vi "Pump Settings Dialog.vi"(8 "error in (no error)":errorcluster, 10 "Message Queues":T15, 11 "Pump Module State Cluster In":T1={"Pump Module Config"={"GUID"="", "Drop Coords"={"Horizontal"=0, "Vertical"=0}, "Process Name"="", "Queue Name"="", "Settings"={"Cycle Period"=500.0, "Ismatech"={"VISA resource name"="", "Simulated?"=TRUE, "Pump Number"=1.0, "Reverse?"=FALSE}, "Masterflex"={"VISA resource name"="", "Simulated?"=TRUE, "Pump Number"=1.0, "Reverse?"=FALSE}, "Manual Entry"=0.0, "VICI Settings"={"VISA resource name"="", "Simulated?"=TRUE, "Pump Letter"="", "Reverse?"=FALSE}, "Output Device"=enum."Default", "Tacmina Settings"={"Analog DAQ Task"="", "Digital DAQ Task"=""}, "KNF SIMDOS Settings"={"VISA resource name"="", "Simulated?"=TRUE}, "ASIA Pump C"={"ASIA Pump #"=0, "channel"=0, "Simulated"=FALSE}, "FLOM Settings"={"VISA resource name"="", "Simulated?"=TRUE, "Pump Number"=0.0}, "Pump Calibration File"=path "", "Calibration Slope"=0.0, "Calibration Y Intercept"=0.0, "Pump Cal Enum"=0, "SSI PR Settings"={"VISA resource name"="", "Simulated?"=FALSE}}, "Load Count"=0}, "State"=enum."Idle", "Start Time"=timestamp(0 s since 1904-01-01), "Current Time"=timestamp(0 s since 1904-01-01), "First Iteration"=FALSE, "Data"={"Pump Speed"=0.0}, "Process Name"="", "Pump On?"=FALSE} {"Pump Module Config"."Settings"."ASIA Pump C"."channel" min=0 max=1 step=1; "Pump Module Config"."Settings"."Masterflex"."Pump Number" min=1.0 max=20.0 step=1.0; "Pump Module Config"."Settings"."Ismatech"."Pump Number" min=1.0 max=20.0 step=1.0}) -> (0 "error out":errorcluster, 1 "Cancelled?":bool=TRUE, 2 "UI Refresh Needed?":bool, 3 "Pump Module Config Out":T2={"GUID"="", "Drop Coords"={"Horizontal"=0, "Vertical"=0}, "Process Name"="", "Queue Name"="", "Settings"={"Cycle Period"=0.0, "Ismatech"={"VISA resource name"="", "Simulated?"=FALSE, "Pump Number"=0.0, "Reverse?"=FALSE}, "Masterflex"={"VISA resource name"="", "Simulated?"=FALSE, "Pump Number"=0.0, "Reverse?"=FALSE}, "Manual Entry"=0.0, "VICI Settings"={"VISA resource name"="", "Simulated?"=FALSE, "Pump Letter"="", "Reverse?"=FALSE}, "Output Device"=enum."Default", "Tacmina Settings"={"Analog DAQ Task"="", "Digital DAQ Task"=""}, "KNF SIMDOS Settings"={"VISA resource name"="", "Simulated?"=TRUE}, "ASIA Pump C"={"ASIA Pump #"=0, "channel"=0, "Simulated"=FALSE}, "FLOM Settings"={"VISA resource name"="", "Simulated?"=TRUE, "Pump Number"=0.0}, "Pump Calibration File"=path "", "Calibration Slope"=0.0, "Calibration Y Intercept"=0.0, "Pump Cal Enum"=0, "SSI PR Settings"={"VISA resource name"="", "Simulated?"=FALSE}}, "Load Count"=0} {"Settings"."ASIA Pump C"."channel" min=0 max=1 step=1; "Settings"."Masterflex"."Pump Number" min=1.0 max=20.0 step=1.0; "Settings"."Ismatech"."Pump Number" min=1.0 max=20.0 step=1.0})   [LabVIEW 2018, in "Pump Module.lvlib"]
doc: "Dialog for selecting user specified settings."
uses:
  Pump Module.lvlib
  Settings/Settings.lvlib
  support/Support Library.lvlib
  Masterflex 7550-30/Masterflex 7550-30.lvlib
  Ismatec ISM 831C/Ismatec ISM 831C.lvlib
  Tacmina QI/Tacmina QI.lvlib
  KNF Pump/KNF SIMDOS.lvlib
  VICI M50 Party Mode/VICI M50 Party Mode.lvlib
  support/Message Queue/Message Queue.lvlib
  support/Message Queue/Enqueue Message (Single).vi
  FLOM Pump/FLOM Pump.lvlib
  SSI PR Class/SSI PR Pump.lvlib
  Measure Instrument/PID 2 Output Enum.ctl
  <vilib>/Utility/xml.llb/Write to XML File(string).vi
  <vilib>/Utility/file.llb/Read Delimited Spreadsheet (string).vi
  Ismatec ISM 831C/Controls/Ismatech Settings Cluster.ctl
  Masterflex 7550-30/Controls/Settings Cluster.ctl
  <vilib>/Utility/miscctls.llb/LVPoint32TypeDef.ctl
  Pump Module Settings Cluster.ctl
  Pump Module Config Cluster.ctl
  support/Message Queue/Message Cluster.ctl
  All Message Queues.ctl
  Tacmina QI/Tacmina QI DAQ Setting.ctl
  Measure Instrument/State Enum.ctl
  Measure Instrument/Feed Module Engine.lvlib
  Pump Module State Cluster.ctl
  KNF Pump/Settings Cluster plus SIMDOS.ctl
  ASIA Pump/Pump Settings.ctl
  ASIA Pump.lvlib
  VICI M50 Party Mode/Settings Cluster.ctl
  FLOM Pump/Settings Cluster.ctl
  SSI PR Class/SSI PR Settings Cluster.ctl
panel:
  in  "Module Name":string
  out "FLOM VISA Chosen":bool
  out "FLOM Number Chosen":bool
  in  "Pump Settings":T16={"Pump Configuration"={"Cycle Period"=500.0, "Ismatech"={"VISA resource name"="", "Simulated?"=FALSE, "Pump Number"=1.0, "Reverse?"=FALSE}, "Masterflex"={"VISA resource name"="", "Simulated?"=FALSE, "Pump Number"=1.0, "Reverse?"=FALSE}, "Pump %"=0.0, "VICI Settings"={"VISA resource name"="", "Simulated?"=FALSE, "Pump Letter"="", "Reverse?"=FALSE}, "Output Device"=enum."Default", "Tacmina Settings"={"Analog DAQ Task"="", "Digital DAQ Task"=""}, "KNF SIMDOS Settings"={"VISA resource name"="", "Simulated?"=FALSE}, "ASIA Pump C"={"ASIA Pump #"=-1, "channel"=-1, "Simulated"=FALSE}, "FLOM Settings"={"VISA resource name"="", "Simulated?"=FALSE, "Pump Number"=1.0}, "Pump Calibration"=0, "SSI PR Settings"={"VISA resource name"="", "Simulated?"=FALSE}}, "Stop"=FALSE, "Start"=FALSE} {"Pump Configuration"."ASIA Pump C"."channel" min=-1 max=1 step=1; "Pump Configuration"."Ismatech"."Pump Number" min=1.0 max=20.0 step=1.0; "Pump Configuration"."Masterflex"."Pump Number" min=1.0 max=20.0 step=1.0}
  in  "Cancel Button":bool
  in  "OK Button":bool
  # "Non visible portion of dialog (needed for connector pane)."
  # "Output Instruments"
  # "Output Instruments"
  # "Output Instruments"
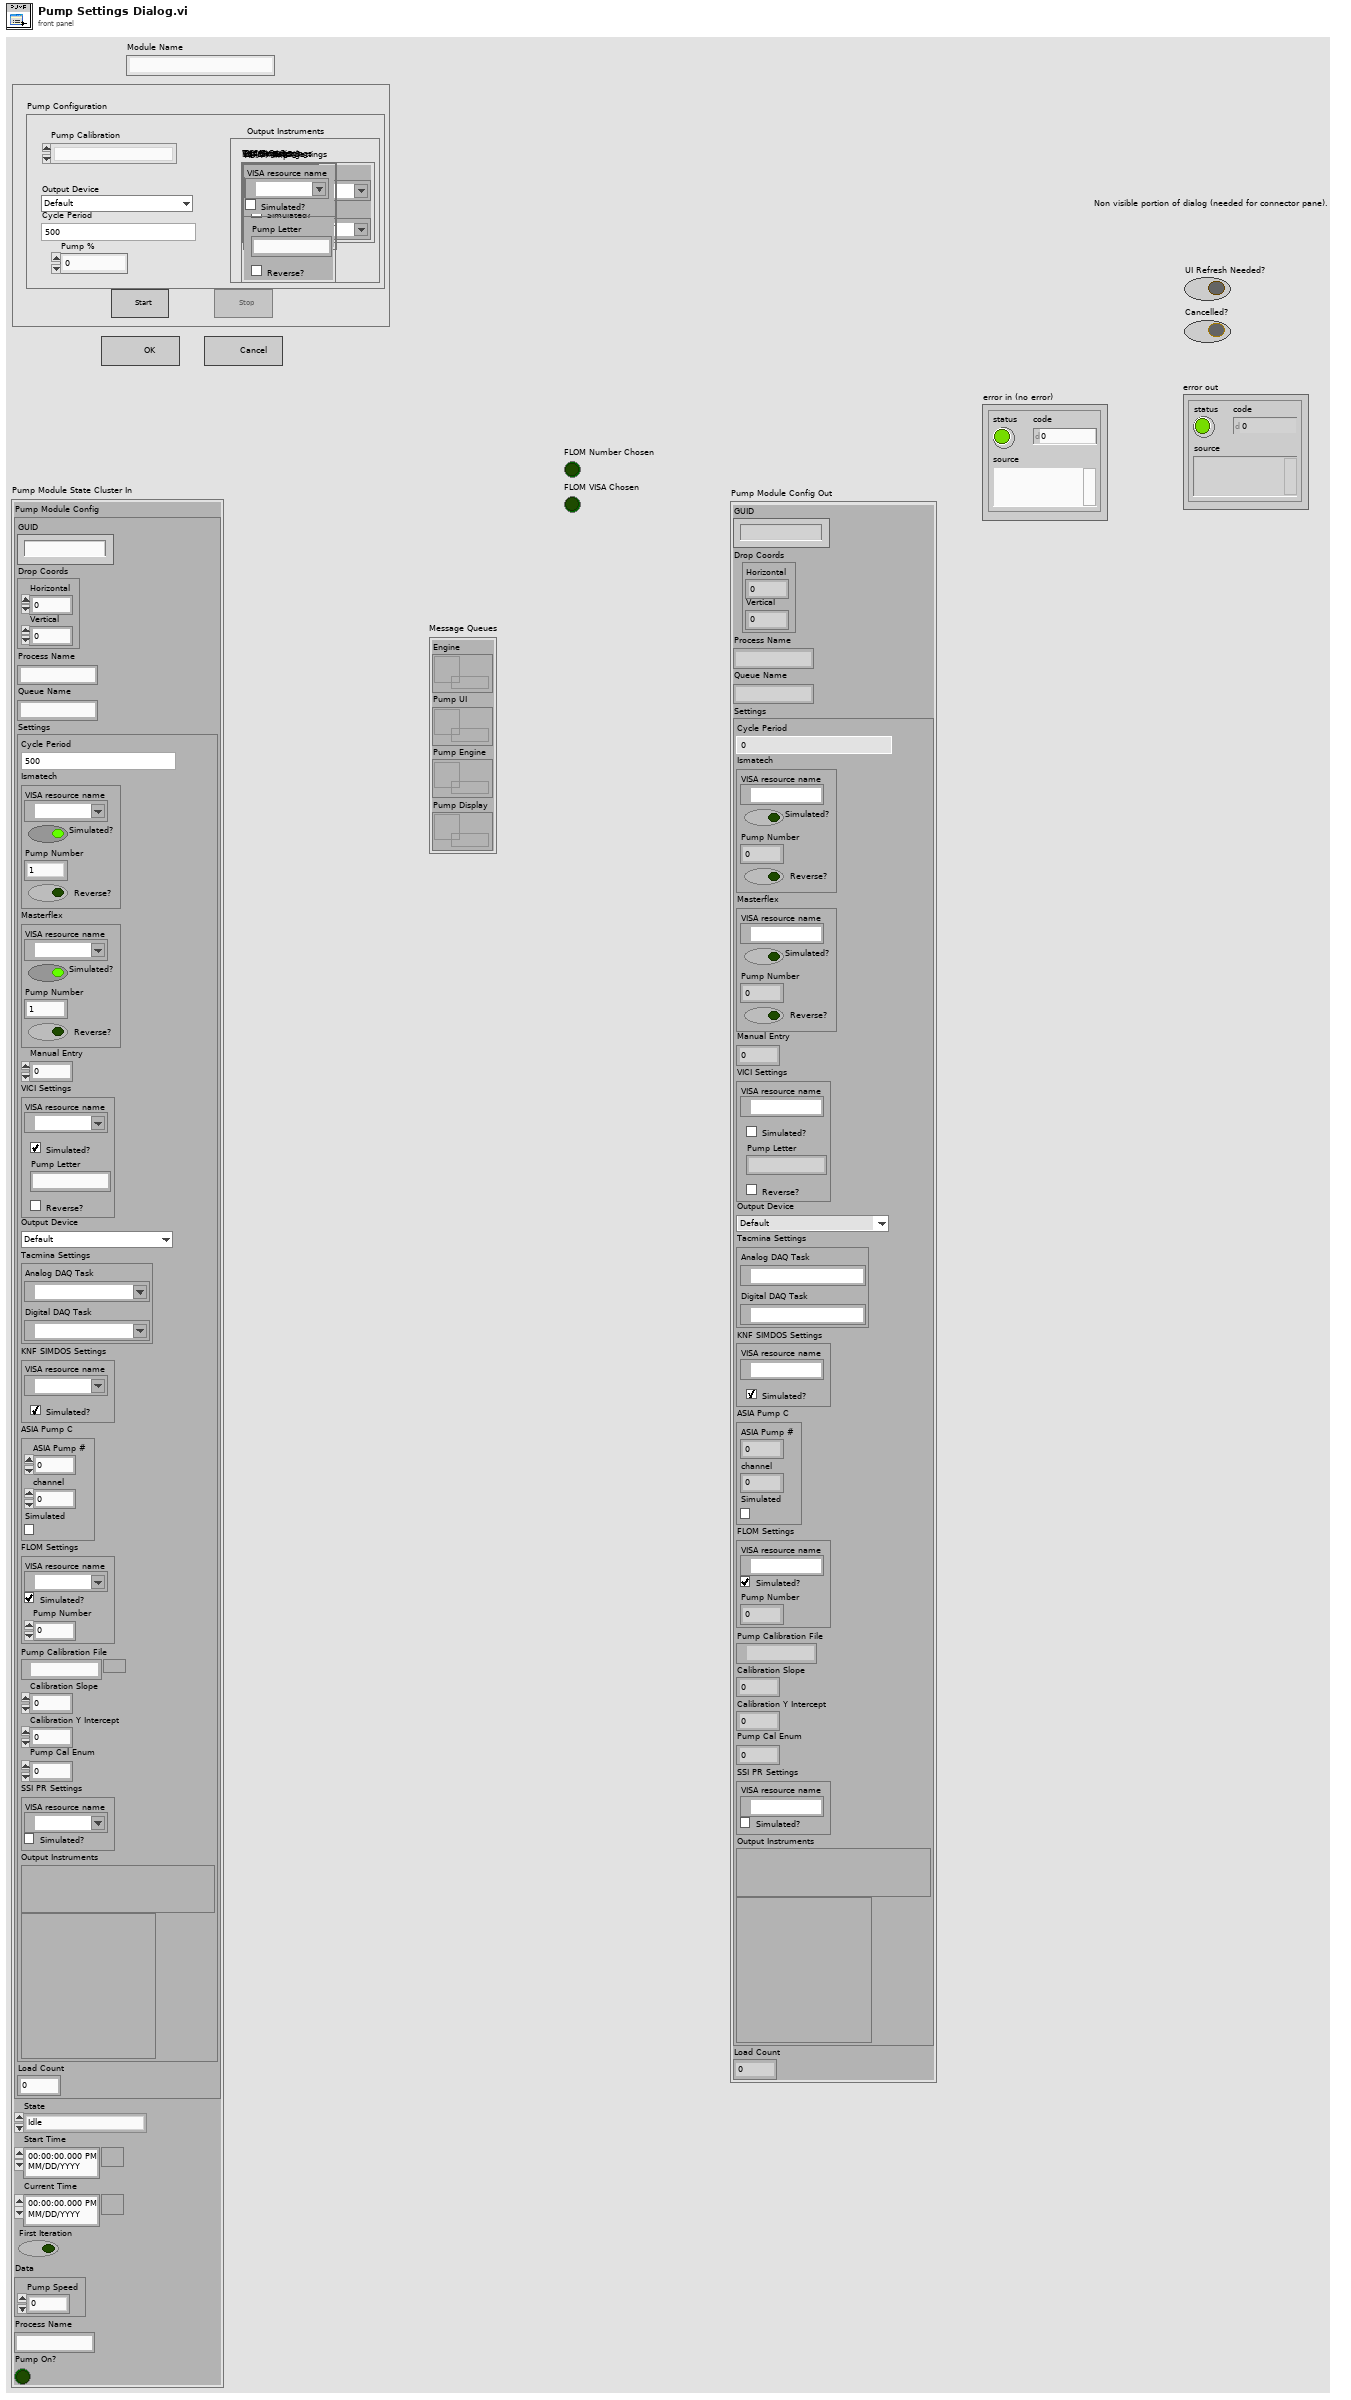
[diagram p1: front panel]
types:
  T1 = typedef "Pump Module.lvlib/Pump Module State Cluster.ctl" = cluster{"Pump Module Config":T2, "State":T14, "Start Time":timestamp, "Current Time":timestamp, "First Iteration":bool, "Data":cluster{"Pump Speed":dbl}, "Process Name":string, "Pump On?":bool}
  T2 = typedef "Pump Module.lvlib/Pump Module Config Cluster.ctl" = cluster{"GUID":string, "Drop Coords":T3, "Process Name":string, "Queue Name":string, "Settings":T4, "Load Count":i32}
  T3 = typedef "LVPoint32TypeDef.ctl" = cluster{"Horizontal":i32, "Vertical":i32}
  T4 = typedef "Pump Module.lvlib/Pump Module Settings Cluster.ctl" = cluster{"Cycle Period":dbl, "Ismatech":T5, "Masterflex":T6, "Manual Entry":dbl, "VICI Settings":T7, "Output Device":T8, "Tacmina Settings":T9, "KNF SIMDOS Settings":T10, "ASIA Pump C":T11, "FLOM Settings":T12, "Pump Calibration File":path, "Calibration Slope":dbl, "Calibration Y Intercept":dbl, "Pump Cal Enum":u16, "SSI PR Settings":T13}
  T5 = typedef "Ismatec ISM 831C.lvlib/Ismatech Settings Cluster.ctl" = cluster{"VISA resource name":refnum<visa-resource-name>, "Simulated?":bool, "Pump Number":dbl, "Reverse?":bool}
  T6 = typedef "Masterflex 7550-30.lvlib/Settings Cluster.ctl" = cluster{"VISA resource name":refnum<visa-resource-name>, "Simulated?":bool, "Pump Number":dbl, "Reverse?":bool}
  T7 = typedef "VICI M50 Party Mode.lvlib/Settings Cluster.ctl" = cluster{"VISA resource name":refnum<visa-resource-name>, "Simulated?":bool, "Pump Letter":string, "Reverse?":bool}
  T8 = typedef "PID 2 Output Enum.ctl" = enum16{"Default", "Ismatec ISM 831C", "Masterflex 7550-30", "VICI", "Tacmina QI", "KNF SIMDOS", "ASIA Type C", "FLOM UI-22-11", "SSI PR"}
  T9 = typedef "Tacmina QI.lvlib/Tacmina QI DAQ Setting.ctl" = cluster{"Analog DAQ Task":refnum<k21>, "Digital DAQ Task":refnum<k21>}
  T10 = typedef "KNF SIMDOS.lvlib/Settings Cluster plus SIMDOS.ctl" = cluster{"VISA resource name":refnum<visa-resource-name>, "Simulated?":bool}
  T11 = typedef "ASIA Pump.lvlib/Pump Settings.ctl" = cluster{"ASIA Pump #":i32, "channel":i32, "Simulated":bool}
  T12 = typedef "FLOM Pump.lvlib/Settings Cluster.ctl" = cluster{"VISA resource name":refnum<visa-resource-name>, "Simulated?":bool, "Pump Number":dbl}
  T13 = typedef "SSI PR Pump.lvlib/SSI PR Settings Cluster.ctl" = cluster{"VISA resource name":refnum<visa-resource-name>, "Simulated?":bool}
  T14 = typedef "Feed Module.lvlib/Feed Module Engine.lvlib/State Enum.ctl" = enum16{"Measuring", "Idle", "Paused"}
  T15 = typedef "Pump Module.lvlib/All Message Queues.ctl" = cluster{"Engine":refnum<queue>, "Pump UI":refnum<queue>, "Pump Engine":refnum<queue>, "Pump Display":refnum<queue>}
  T16 = cluster{"Pump Configuration":cluster{"Cycle Period":dbl, "Ismatech":T5, "Masterflex":T6, "Pump %":dbl, "VICI Settings":T7, "Output Device":T8, "Tacmina Settings":T9, "KNF SIMDOS Settings":T10, "ASIA Pump C":T11, "FLOM Settings":T12, "Pump Calibration":u16, "SSI PR Settings":T13}, "Stop":bool, "Start":bool}
  T17 = enum8{"Enabled", "Disabled", "Disabled and Grayed Out"}
  T18 = typedef "VICI M6 M50 Party Mode.lvlib/Settings Cluster.ctl" = cluster{"VISA resource name":refnum<visa-resource-name>, "Simulated?":bool, "Pump Letter":string, "Reverse?":bool}
  T19 = cluster{"Cycle Period":dbl, "Ismatech":T5, "Masterflex":T6, "Pump %":dbl, "VICI Settings":T18, "Output Device":T8, "Tacmina Settings":T9, "KNF SIMDOS Settings":T10, "ASIA Pump C":T11, "FLOM Settings":T12, "Pump Calibration":u16, "SSI PR Settings":T13}
  T20 = cluster{"Cycle Period":dbl, "Ismatech":T5, "Masterflex":T6, "Pump %":dbl, "VICI Settings":T7, "Output Device":T8, "Tacmina Settings":T9, "KNF SIMDOS Settings":T10, "ASIA Pump C":T11, "FLOM Settings":T12, "Pump Calibration":u16, "SSI PR Settings":T13}
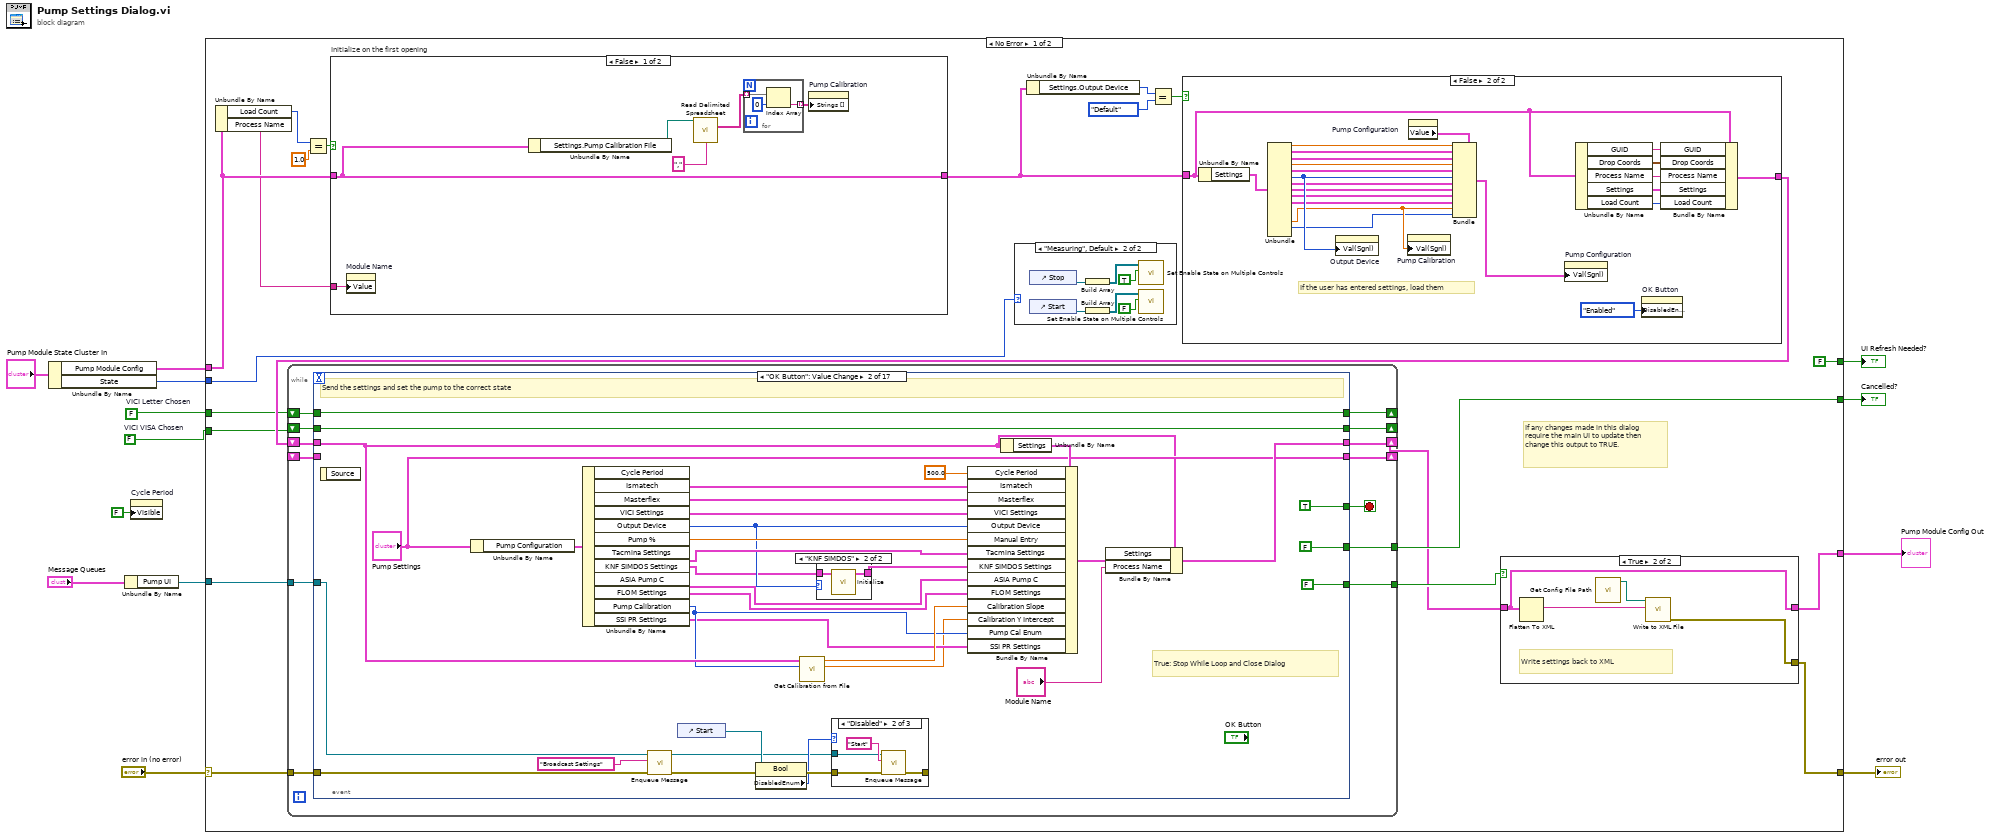
[diagram p0: block diagram]
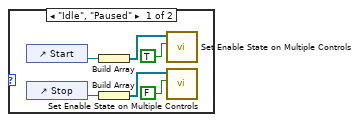
[diagram p2: hidden frame]
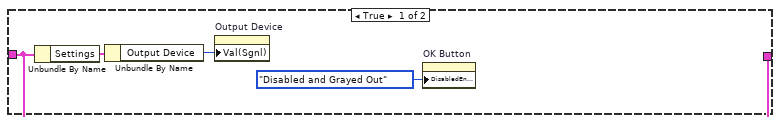
[diagram p3: hidden frame]
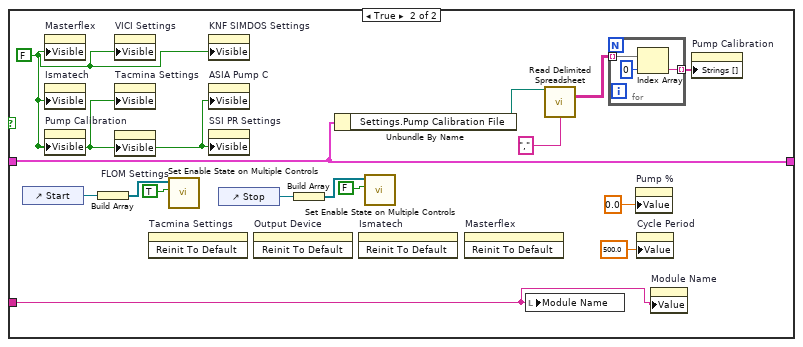
[diagram p4: hidden frame]
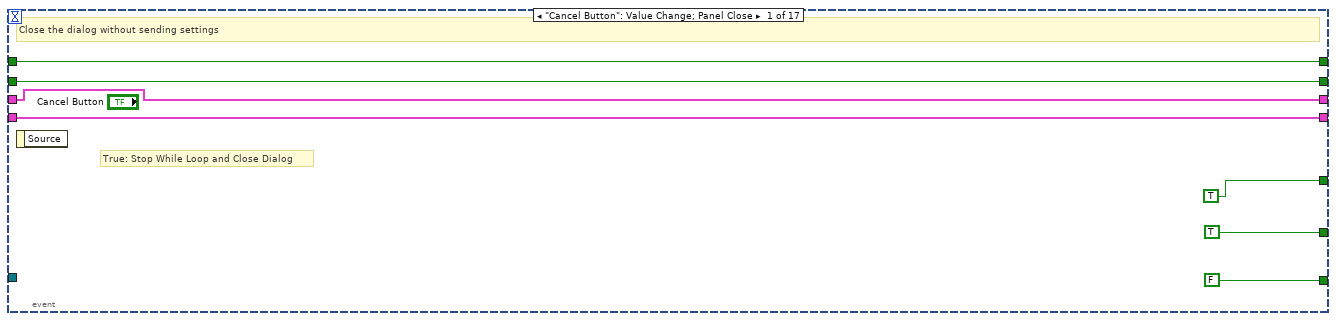
[diagram p5: hidden frame]
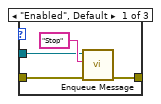
[diagram p6: hidden frame]
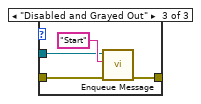
[diagram p7: hidden frame]
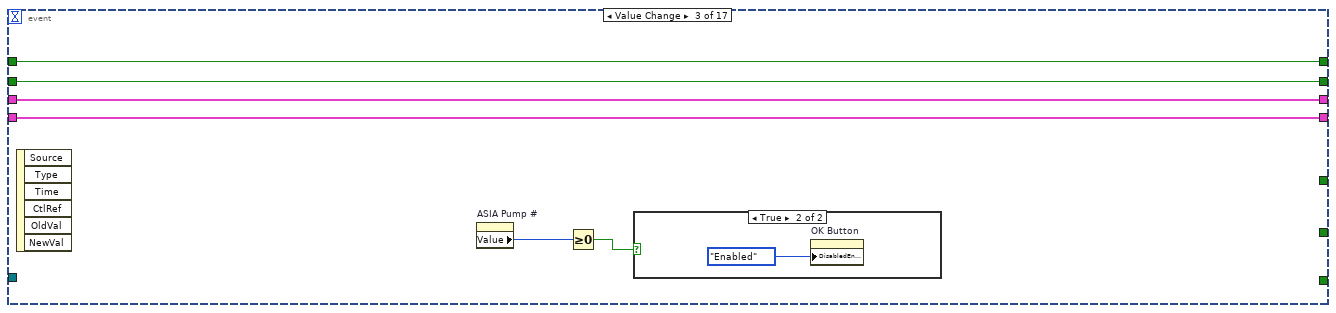
[diagram p9: hidden frame]
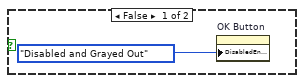
[diagram p10: hidden frame]
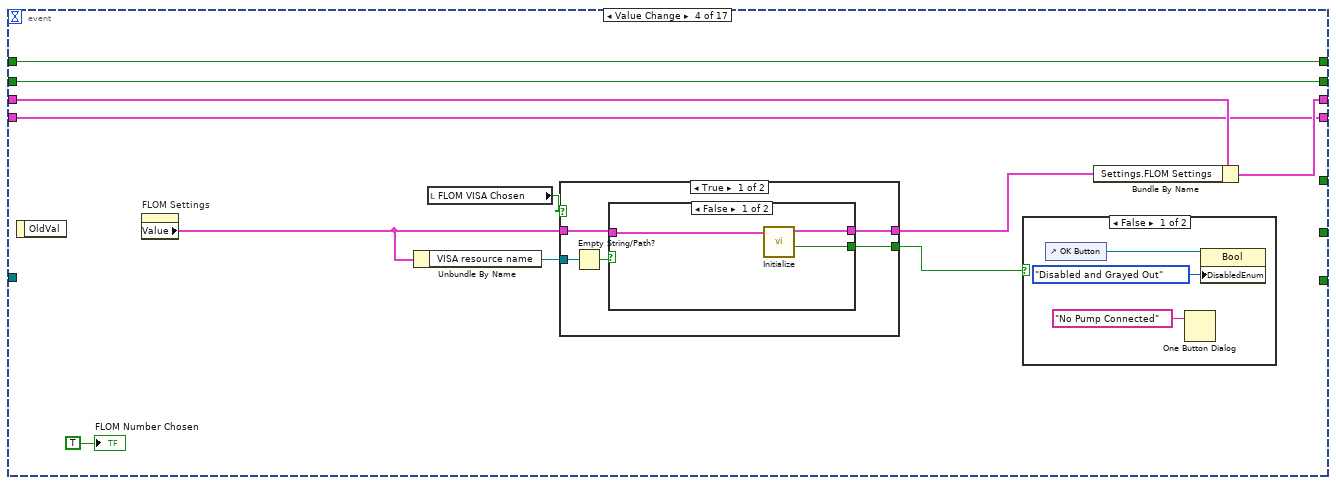
[diagram p11: hidden frame]
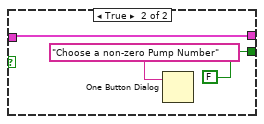
[diagram p12: hidden frame]
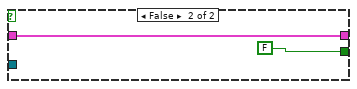
[diagram p13: hidden frame]
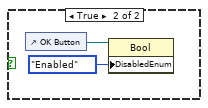
[diagram p14: hidden frame]
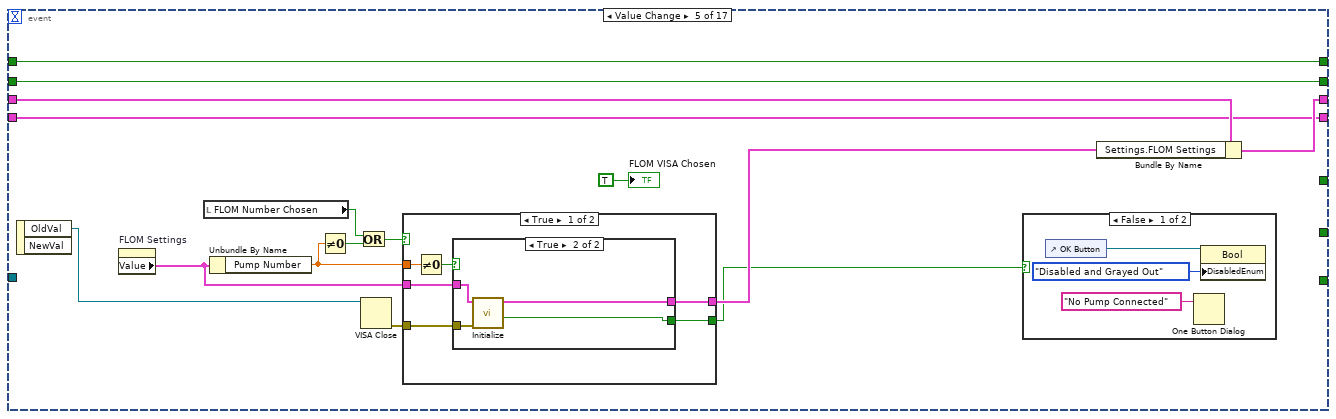
[diagram p15: hidden frame]
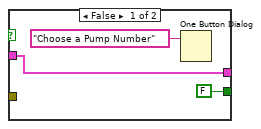
[diagram p16: hidden frame]
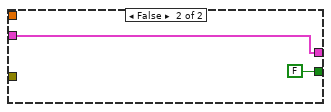
[diagram p17: hidden frame]
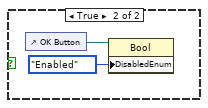
[diagram p18: hidden frame]
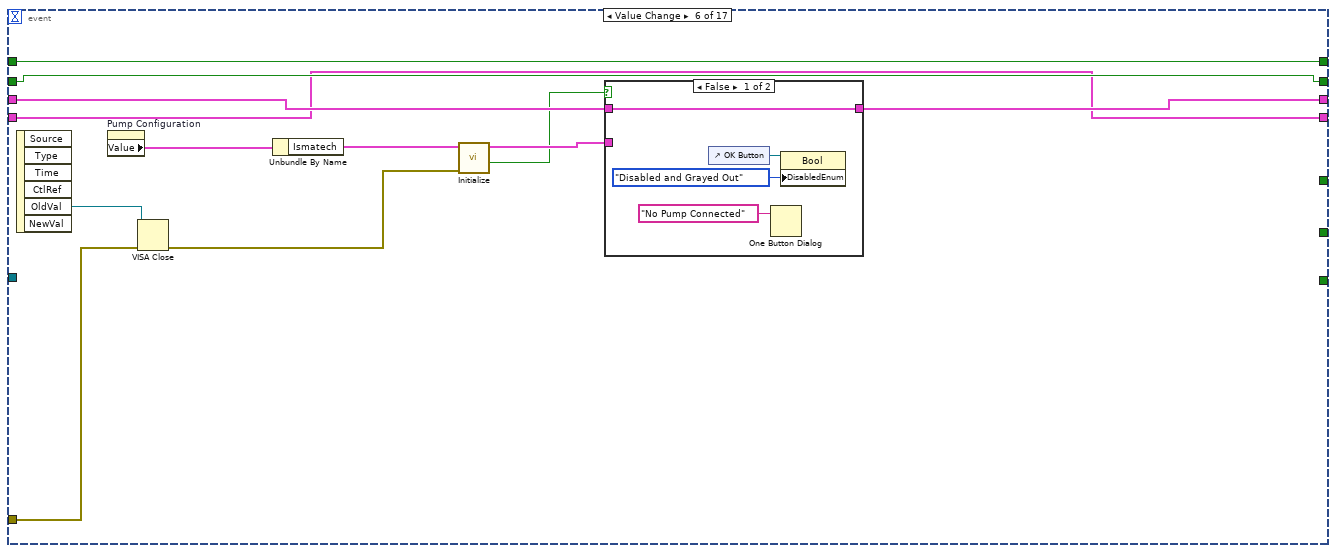
[diagram p19: hidden frame]
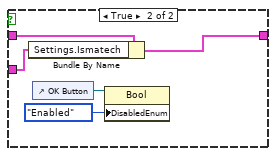
[diagram p20: hidden frame]
diagram:
  w2 = FALSE  # VICI VISA Chosen
  w3 = FALSE  # VICI Letter Chosen
  n1 = Unbundle By Name("Pump Module State Cluster In") -> ("Pump Module Config"=w5:T2, "State"=w4:T14)
  n2 = Unbundle By Name("Message Queues") -> ("Pump UI"=w10:refnum<queue>)
  n3 = property on="Cycle Period" class="DigNum (strict)"("Visible"=FALSE) -> ()  [unwired: 2 in, 2 out]
  n4 = case shown="No Error" "error in (no error)" {
    selector: "error in (no error)" -> [w29 w534]
    tunnel: [w31 w534] -> w13
    tunnel: w5 -> [w28 w532]
    tunnel: [w32 w532] -> w7
    tunnel: [FALSE ("UI Refresh Needed?") _] -> w12
    tunnel: [w33 TRUE ("UI Refresh Needed?")] -> w11
    tunnel: w10 -> [w30 _]
    tunnel: w4 -> [w27 _]
    tunnel: w3 -> [w20 _]
    tunnel: w2 -> [w19 _]
    frame No Error {
      # "If any changes made in this dialog require the main UI to update then change this output to TRUE."
      n5 = Unbundle By Name(w28) -> ("Load Count"=w26:i32, "Process Name"=w14:string)
      n6 = Equal?(x=w26, y=1.0) -> (x = y?=w24:bool)
      n7 = case "Initialize on the first opening" shown="False" w24 {
        tunnel: w28 -> [w75 w97]
        tunnel: [w75 w97] -> w18
        tunnel: w14 -> [w74 w83]
        frame False {
          n8 = property on="Module Name" class="Str"("Value"=w74) -> ()  [unwired: 2 in, 2 out]
          n9 = Unbundle By Name(w75) -> ("Settings.Pump Calibration File"=w79:path)
          n10 = call-poly <vilib>:"Read Delimited Spreadsheet.vi"("file path (dialog if empty)"=w79, "delimiter (\\t)"="," ("delimiter (\\t)")) -> ("all rows"=w78:string[][])  [unwired: 8 in, 5 out]
          n11 = for {
            tunnel: w78 -> [w81] mode=indexing
            tunnel: [w80] -> w77 mode=indexing
            n12 = Index Array(array=w81, index=0) -> (element=w80:string)
          }
          n13 = property on="Pump Calibration" class="Ring (strict)"("Strings []"=w77) -> ()  [unwired: 2 in, 2 out]
        }
        frame True {
          w84 = FALSE ("Visible")
          n14 = control-ref of="Start"() -> (w91:refnum<vi>)
          n15 = property on="Masterflex" class="Clust (strict)"("Visible"=w84) -> ()  [unwired: 2 in, 2 out]
          n16 = property on="Ismatech" class="Clust (strict)"("Visible"=w84) -> ()  [unwired: 2 in, 2 out]
          n17 = property on="Pump Calibration" class="Ring (strict)"("Visible"=w84) -> ()  [unwired: 2 in, 2 out]
          n18 = Build Array(w91) -> (w92:refnum<vi>[])
          n19 = property on="VICI Settings" class="Clust (strict)"("Visible"=w84) -> ()  [unwired: 2 in, 2 out]
          n20 = property on="Tacmina Settings" class="Clust (strict)"("Visible"=w84) -> ()  [unwired: 2 in, 2 out]
          n21 = property on="FLOM Settings" class="Clust (strict)"("Visible"=w84) -> ()  [unwired: 2 in, 2 out]
          n22 = invoke on="Tacmina Settings" class="Clust (strict)" method="Reinit To Default"() -> ()  [unwired: 3 in, 3 out]
          n23 = call "Set Enable State on Multiple Controls.vi"("Enable?"=TRUE, "Controls"=w92) -> ()  [unwired: 10 in]
          n24 = property on="KNF SIMDOS Settings" class="Clust (strict)"("Visible"=w84) -> ()  [unwired: 2 in, 2 out]
          n25 = property on="ASIA Pump C" class="Clust (strict)"("Visible"=w84) -> ()  [unwired: 2 in, 2 out]
          n26 = property on="SSI PR Settings" class="Clust (strict)"("Visible"=w84) -> ()  [unwired: 2 in, 2 out]
          n27 = control-ref of="Stop"() -> (w94:refnum<vi>)
          n28 = invoke on="Output Device" class="Enum (strict)" method="Reinit To Default"() -> ()  [unwired: 3 in, 3 out]
          n29 = Build Array(w94) -> (w95:refnum<vi>[])
          n30 = Unbundle By Name(w97) -> ("Settings.Pump Calibration File"=w88:path)
          n31 = invoke on="Ismatech" class="Clust (strict)" method="Reinit To Default"() -> ()  [unwired: 3 in, 3 out]
          n32 = call "Set Enable State on Multiple Controls.vi"("Enable?"=FALSE, "Controls"=w95) -> ()  [unwired: 10 in]
          n33 = invoke on="Masterflex" class="Clust (strict)" method="Reinit To Default"() -> ()  [unwired: 3 in, 3 out]
          n34 = local write "Module Name"(w83) -> ()
          n35 = call-poly <vilib>:"Read Delimited Spreadsheet.vi"("file path (dialog if empty)"=w88, "delimiter (\\t)"="," ("delimiter (\\t)")) -> ("all rows"=w86:string[][])  [unwired: 8 in, 5 out]
          n36 = for {
            tunnel: w86 -> [w99] mode=indexing
            tunnel: [w98] -> w85 mode=indexing
            n37 = Index Array(array=w99, index=0) -> (element=w98:string)
          }
          n38 = property on="Pump %" class="DigNum (strict)"("Value"=0.0) -> ()  [unwired: 2 in, 2 out]
          n39 = property on="Cycle Period" class="DigNum (strict)"("Value"=500.0) -> ()  [unwired: 2 in, 2 out]
          n40 = property on="Module Name" class="Str"("Value"=w83) -> ()  [unwired: 2 in, 2 out]
          n41 = property on="Pump Calibration" class="Ring (strict)"("Strings []"=w85) -> ()  [unwired: 2 in, 2 out]
        }
      }
      n42 = case shown="\"Measuring\", Default" w27 {
        frame "Idle", "Paused" {
          n43 = control-ref of="Start"() -> (w35:refnum<vi>)
          n44 = control-ref of="Stop"() -> (w37:refnum<vi>)
          n45 = Build Array(w35) -> (w39:refnum<vi>[])
          n46 = Build Array(w37) -> (w36:refnum<vi>[])
          n47 = call "Set Enable State on Multiple Controls.vi"("Enable?"=TRUE, "Controls"=w39) -> ()  [unwired: 10 in]
          n48 = call "Set Enable State on Multiple Controls.vi"("Enable?"=FALSE, "Controls"=w36) -> ()  [unwired: 10 in]
        }
        frame "Measuring", Default {
          n49 = control-ref of="Stop"() -> (w41:refnum<vi>)
          n50 = control-ref of="Start"() -> (w42:refnum<vi>)
          n51 = Build Array(w41) -> (w45:refnum<vi>[])
          n52 = Build Array(w42) -> (w43:refnum<vi>[])
          n53 = call "Set Enable State on Multiple Controls.vi"("Enable?"=TRUE, "Controls"=w45) -> ()  [unwired: 10 in]
          n54 = call "Set Enable State on Multiple Controls.vi"("Enable?"=FALSE, "Controls"=w43) -> ()  [unwired: 10 in]
        }
      }
      n55 = Unbundle By Name(w18) -> ("Settings.Output Device"=w16:T8)
      n56 = Equal?(x=w16, y=PID_2_Output_Enum."Default" ("Settings.Output Device")) -> (x = y?=w15:bool)
      n57 = case shown="False" w15 {
        tunnel: w18 -> [w48 w58]
        tunnel: [w48 w61] -> w21
        frame True {
          n58 = Unbundle By Name(w48) -> ("Settings"=w50:T4)
          n59 = Unbundle By Name(w50) -> ("Output Device"=w49:T8)
          n60 = property on="Output Device" class="Enum (strict)"("Val(Sgnl)"=w49) -> ()  [unwired: 2 in, 2 out]
          n61 = property on="OK Button" class="Bool"("DisabledEnum"=T17."Disabled and Grayed Out" ("Disabled")) -> ()  [unwired: 2 in, 2 out]
        }
        frame False {
          # "If the user has entered settings, load them"
          n62 = Unbundle By Name(w58) -> ("Settings"=w60:T4)
          n63 = Unbundle(w60) -> ("Cycle Period"=w73:dbl, "Ismatech"=w72:T5, "Masterflex"=w71:T6, "Manual Entry"=w70:dbl, "VICI Settings"=w67:T7, "Output Device"=w69:T8, "Tacmina Settings"=w59:T9, "KNF SIMDOS Settings"=w57:T10, "ASIA Pump C"=w56:T11, "FLOM Settings"=w55:T12, "Calibration Y Intercept"=w53:dbl, "Pump Cal Enum"=w51:u16)  [unwired: 3 out]
          n64 = property on="Output Device" class="Enum (strict)"("Val(Sgnl)"=w69) -> ()  [unwired: 2 in, 2 out]
          n65 = property on="Pump Calibration" class="Ring (strict)"("Val(Sgnl)"=w53) -> ()  [unwired: 2 in, 2 out]
          n66 = property on="Pump Configuration" class="Clust (strict)"() -> ("Value"=w52:T19)  [unwired: 2 in, 2 out]
          n67 = Bundle(cluster=w52, "Cycle Period"=w73, "Ismatech"=w72, "Masterflex"=w71, "Pump %"=w70, "VICI Settings"=w67, "Output Device"=w69, "Tacmina Settings"=w59, "KNF SIMDOS Settings"=w57, "ASIA Pump C"=w56, "FLOM Settings"=w55, "Pump Calibration"=w53, "SSI PR Settings"=w51) -> (w68:T19)
          n68 = property on="Pump Configuration" class="Clust (strict)"("Val(Sgnl)"=w68) -> ()  [unwired: 2 in, 2 out]
          n69 = Unbundle By Name(w58) -> ("GUID"=w66:string, "Drop Coords"=w65:T3, "Process Name"=w64:string, "Settings"=w63:T4, "Load Count"=w62:i32)
          n70 = property on="OK Button" class="Bool"("DisabledEnum"=T17."Enabled" ("Disabled")) -> ()  [unwired: 2 in, 2 out]
          n71 = Bundle By Name(cluster=w58, "GUID"=w66, "Drop Coords"=w65, "Process Name"=w64, "Settings"=w63, "Load Count"=w62) -> (w61:T2)
        }
      }
      n72 = while {
        tunnel: [w113] -> w23
        tunnel: [w111] -> w33
        tunnel: w30 -> [w109]
        tunnel: w29 -> [w108]
        shift-right: [w110] -> w22
        shift-left: w21 -> [w107]
        shift-right: [w106] -> _
        shift-left: w20 -> [w105]
        shift-right: [w104] -> _
        shift-left: w19 -> [w103]
        shift-right: [w102] -> _
        shift-left: _ -> [w101]
        stop <- w112 stop-if-true
        n73 = event shown="[1] \"OK Button\": Value Change" {
          selector: _ -> [_ _ _ _ _ _ _ _ _ _ _ _ _ _ _ _ _]
          dyn-events: _ -> [_ _ _ _ _ _ _ _ _ _ _ _ _ _ _ _ _]
          timeout: _ -> [_ _ _ _ _ _ _ _ _ _ _ _ _ _ _ _ _]
          tunnel: [FALSE ("UI Refresh Needed?") FALSE ("UI Refresh Needed?") _ _ _ _ _ _ _ _ _ _ _ _ _ _ _] -> w113
          tunnel: [TRUE TRUE _ _ _ _ _ _ _ _ _ _ _ _ _ _ _] -> w112
          tunnel: [TRUE ("UI Refresh Needed?") FALSE ("UI Refresh Needed?") _ _ _ _ _ _ _ _ _ _ _ _ _ _ _] -> w111
          tunnel: w107 -> [w117 w125 w172 w189 w222 w249 w273 w291 w310 w422 w439 w447 w467 w478 w500 w512 w525]
          tunnel: [w117 w149 w172 w188 w221 w248 w272 w290 w309 w421 w438 w446 w467 w477 w500 w512 w525] -> w110
          tunnel: w109 -> [_ w151 _ _ _ _ _ _ _ _ _ _ _ _ _ _ _]
          tunnel: w108 -> [_ w148 _ _ _ w247 w271 w289 _ w420 _ w445 _ w476 _ _ _]
          tunnel: [w115 w136 w176 w187 w220 w245 w266 w287 w307 TRUE ("VICI VISA Chosen") w436 TRUE ("VICI VISA Chosen") TRUE ("VICI VISA Chosen") w475 w501 w510 w523] -> w106
          tunnel: w105 -> [w115 w136 w176 w187 w220 w245 w266 w287 w307 _ w436 _ _ w475 w501 w510 w523]
          tunnel: [w116 w137 w175 w186 w219 w246 w267 w288 w308 w419 w435 w444 w470 TRUE ("VICI VISA Chosen") w502 w511 w524] -> w104
          tunnel: w103 -> [w116 w137 w175 w186 w219 w246 w267 w288 w308 w419 w435 w444 w470 _ w502 w511 w524]
          tunnel: [w114 "Pump Settings" w174 w185 w218 w244 w265 w286 w306 w417 w434 w442 w468 w473 w499 w509 w522] -> w102
          tunnel: w101 -> [w114 _ w174 w185 w218 w244 w265 w286 w306 w417 w434 w442 w468 w473 w499 w509 w522]
          event "Cancel Button": Value Change; Panel Close {
            # "True: Stop While Loop and Close Dialog"
            # "Close the dialog without sending settings"
            n74 = event-data() -> ()  [unwired: 1 in, 1 out]
          }
          event "OK Button": Value Change {
            # "True: Stop While Loop and Close Dialog"
            # "Send the settings and set the pump to the correct state"
            n75 = event-data() -> ()  [unwired: 1 in, 1 out]
            n76 = Unbundle By Name("Pump Settings") -> ("Pump Configuration"=w147:T20)
            n77 = Unbundle By Name(w147) -> ("Ismatech"=w146:T5, "Masterflex"=w145:T6, "VICI Settings"=w144:T7, "Output Device"=w141:T8, "Pump %"=w143:dbl, "Tacmina Settings"=w142:T9, "KNF SIMDOS Settings"=w140:T10, "ASIA Pump C"=w138:T11, "FLOM Settings"=w127:T12, "Pump Calibration"=w124:u16, "SSI PR Settings"=w123:T13)  [unwired: 1 out]
            n78 = call-poly "Enqueue Message.vi"("error in (no error)"=w148, "Message"="Broadcast Settings", "Message Queue"=w151) -> ("error out"=w130:errorcluster, "dup Message Queue"=w129:refnum<queue>)  [unwired: 7 in]
            n79 = control-ref of="Start"() -> (w133:refnum<vi>)
            n80 = property class="Bool"(reference=w133, error in=w130) -> (error out=w134:errorcluster, "DisabledEnum"=w132:T17)  [unwired: 1 out]
            n81 = call "Get Calibration from File.vi"("Pump Calibration"=w124, "Pump Module Config"=w125) -> ("Calibration Y Intercept"=w121:dbl, "Calibration Slope"=w126:dbl)  [unwired: 8 in]
            n82 = case shown="\"KNF SIMDOS\"" w141 {
              tunnel: w140 -> [w168 w170]
              tunnel: [w168 w169] -> w139
              frame "Default", Default {
              }
              frame "KNF SIMDOS" {
                n83 = call "Initialize.vi"("KNF Settings"=w170) -> ("KNF Settings"=w169:T10)  [unwired: 7 in, 3 out]
              }
            }
            n84 = case shown="\"Disabled\"" w132 {
              tunnel: w134 -> [w157 w162 w166]
              tunnel: [w159 w161 w165] -> _
              tunnel: w129 -> [w156 w160 w164]
              frame "Enabled", Default {
                n85 = call-poly "Enqueue Message.vi"("error in (no error)"=w157, "Message"="Stop", "Message Queue"=w156) -> ("error out"=w159:errorcluster)  [unwired: 7 in, 1 out]
              }
              frame "Disabled" {
                n86 = call-poly "Enqueue Message.vi"("error in (no error)"=w162, "Message"="Start", "Message Queue"=w160) -> ("error out"=w161:errorcluster)  [unwired: 7 in, 1 out]
              }
              frame "Disabled and Grayed Out" {
                n87 = call-poly "Enqueue Message.vi"("error in (no error)"=w166, "Message"="Start", "Message Queue"=w164) -> ("error out"=w165:errorcluster)  [unwired: 7 in, 1 out]
              }
            }
            n88 = Unbundle By Name(w125) -> ("Settings"=w152:T4)
            n89 = Bundle By Name(cluster=w152, "Cycle Period"=500.0, "Ismatech"=w146, "Masterflex"=w145, "VICI Settings"=w144, "Output Device"=w141, "Manual Entry"=w143, "Tacmina Settings"=w142, "KNF SIMDOS Settings"=w139, "ASIA Pump C"=w138, "FLOM Settings"=w127, "Calibration Slope"=w126, "Calibration Y Intercept"=w121, "Pump Cal Enum"=w124, "SSI PR Settings"=w123) -> (w150:T4)
            n90 = Bundle By Name(cluster=w125, "Settings"=w150, "Process Name"="Module Name") -> (w149:T2)
          }
          event Value Change {
            n91 = event-data() -> ()  [unwired: 1 in, 6 out]
            n92 = property on="ASIA Pump #" class="DigNum (strict)"() -> ("Value"=w171:i32)  [unwired: 2 in, 2 out]
            n93 = Greater Or Equal To 0?(x=w171) -> (x >= 0?=w173:bool)
            n94 = case shown="True" w173 {
              frame False {
                n95 = property on="OK Button" class="Bool"("DisabledEnum"=T17."Disabled and Grayed Out" ("Disabled")) -> ()  [unwired: 2 in, 2 out]
              }
              frame True {
                n96 = property on="OK Button" class="Bool"("DisabledEnum"=T17."Enabled" ("Disabled")) -> ()  [unwired: 2 in, 2 out]
              }
            }
          }
          event Value Change {
            n97 = event-data() -> ()  [unwired: 1 in, 1 out]
            n98 = property on="FLOM Settings" class="Clust (strict)"() -> ("Value"=w182:T12)  [unwired: 2 in, 2 out]
            n99 = Unbundle By Name(w182) -> ("VISA resource name"=w179:refnum<visa-resource-name>)
            n100 = local read "FLOM VISA Chosen"() -> (w180:bool)
            n101 = case shown="True" w180 {
              tunnel: w182 -> [w194 w202]
              tunnel: [w193 w202] -> w184
              tunnel: [w192 FALSE ("Initialized")] -> w183
              tunnel: w179 -> [w190 _]
              frame True {
                n102 = Empty String/Path?(string/path=w190) -> (empty?=w191:bool)
                n103 = case shown="False" w191 {
                  tunnel: w194 -> [w197 w199]
                  tunnel: [w196 w199] -> w193
                  tunnel: [w195 FALSE ("Initialized")] -> w192
                  frame False {
                    n104 = call "Initialize.vi"("FLOM Settings in"=w197) -> ("Initialized"=w195:bool, "FLOM Settings out"=w196:T12)  [unwired: 7 in, 2 out]
                  }
                  frame True {
                    n105 = One Button Dialog(message="Choose a non-zero Pump Number") -> ()  [unwired: 1 in, 1 out]
                  }
                }
              }
              frame False {
              }
            }
            n106 = case shown="False" w183 {
              frame False {
                n107 = control-ref of="OK Button"() -> (w204:refnum<vi>)
                n108 = One Button Dialog(message="No Pump Connected") -> ()  [unwired: 1 in, 1 out]
                n109 = property class="Bool"(reference=w204, "DisabledEnum"=T17."Disabled and Grayed Out" ("Disabled")) -> ()  [unwired: 1 in, 2 out]
              }
              frame True {
                n110 = control-ref of="OK Button"() -> (w206:refnum<vi>)
                n111 = property class="Bool"(reference=w206, "DisabledEnum"=T17."Enabled" ("Disabled")) -> ()  [unwired: 1 in, 2 out]
              }
            }
            n112 = Bundle By Name(cluster=w189, "Settings.FLOM Settings"=w184) -> (w188:T2)
            "FLOM Number Chosen" <- TRUE ("FLOM Number Chosen")
          }
          event Value Change {
            n113 = event-data() -> ("OldVal"=w216:refnum<visa-resource-name>)  [unwired: 1 in, 1 out]
            n114 = property on="FLOM Settings" class="Clust (strict)"() -> ("Value"=w213:T12)  [unwired: 2 in, 2 out]
            n115 = local read "FLOM Number Chosen"() -> (w211:bool)
            n116 = Unbundle By Name(w213) -> ("Pump Number"=w210:dbl)
            n117 = Not Equal To 0?(x=w210) -> (x != 0?=w209:bool)
            n118 = Or(x=w211, y=w209) -> (x .or. y?=w208:bool)
            n119 = VISA Close(VISA resource name=w216) -> (error out=w215:errorcluster)  [unwired: 1 in]
            n120 = case shown="True" w208 {
              tunnel: w213 -> [w228 w237]
              tunnel: [w227 w237] -> w217
              tunnel: w215 -> [w226 _]
              tunnel: [w225 FALSE ("Initialized")] -> w214
              tunnel: w210 -> [w224 _]
              frame True {
                n121 = Not Equal To 0?(x=w224) -> (x != 0?=w223:bool)
                n122 = case shown="True" w223 {
                  tunnel: w228 -> [w230 w235]
                  tunnel: [w230 w234] -> w227
                  tunnel: w226 -> [_ w233]
                  tunnel: [FALSE ("Initialized") w232] -> w225
                  frame False {
                    n123 = One Button Dialog(message="Choose a Pump Number") -> ()  [unwired: 1 in, 1 out]
                  }
                  frame True {
                    n124 = call "Initialize.vi"("error in (no error)"=w233, "FLOM Settings in"=w235) -> ("Initialized"=w232:bool, "FLOM Settings out"=w234:T12)  [unwired: 6 in, 2 out]
                  }
                }
              }
              frame False {
              }
            }
            n125 = case shown="False" w214 {
              frame False {
                n126 = control-ref of="OK Button"() -> (w239:refnum<vi>)
                n127 = One Button Dialog(message="No Pump Connected") -> ()  [unwired: 1 in, 1 out]
                n128 = property class="Bool"(reference=w239, "DisabledEnum"=T17."Disabled and Grayed Out" ("Disabled")) -> ()  [unwired: 1 in, 2 out]
              }
              frame True {
                n129 = control-ref of="OK Button"() -> (w241:refnum<vi>)
                n130 = property class="Bool"(reference=w241, "DisabledEnum"=T17."Enabled" ("Disabled")) -> ()  [unwired: 1 in, 2 out]
              }
            }
            n131 = Bundle By Name(cluster=w222, "Settings.FLOM Settings"=w217) -> (w221:T2)
            "FLOM VISA Chosen" <- TRUE ("FLOM VISA Chosen")
          }
          event Value Change {
            n132 = event-data() -> ("OldVal"=w250:refnum<visa-resource-name>)  [unwired: 1 in, 5 out]
            n133 = property on="Pump Configuration" class="Clust (strict)"() -> ("Value"=w251:T19)  [unwired: 2 in, 2 out]
            n134 = VISA Close(VISA resource name=w250, error in (no error)=w247) -> (error out=w252:errorcluster)
            n135 = Unbundle By Name(w251) -> ("Ismatech"=w254:T5)
            n136 = call "Initialize.vi"("error in (no error)"=w252, "Ismatech Settings"=w254) -> ("Initialized"=w243:bool, "Ismatech Settings"=w253:T5)  [unwired: 6 in, 2 out]
            n137 = case shown="False" w243 {
              tunnel: w253 -> [_ w263]
              tunnel: w249 -> [w258 w259]
              tunnel: [w258 w262] -> w248
              frame False {
                n138 = control-ref of="OK Button"() -> (w256:refnum<vi>)
                n139 = One Button Dialog(message="No Pump Connected") -> ()  [unwired: 1 in, 1 out]
                n140 = property class="Bool"(reference=w256, "DisabledEnum"=T17."Disabled and Grayed Out" ("Disabled")) -> ()  [unwired: 1 in, 2 out]
              }
              frame True {
                n141 = Bundle By Name(cluster=w259, "Settings.Ismatech"=w263) -> (w262:T2)
                n142 = control-ref of="OK Button"() -> (w260:refnum<vi>)
                n143 = property class="Bool"(reference=w260, "DisabledEnum"=T17."Enabled" ("Disabled")) -> ()  [unwired: 1 in, 2 out]
              }
            }
          }
          event Value Change {
            n144 = event-data() -> ("OldVal"=w275:refnum<visa-resource-name>)  [unwired: 1 in, 5 out]
            n145 = property on="Pump Configuration" class="Clust (strict)"() -> ("Value"=w274:T19)  [unwired: 2 in, 2 out]
            n146 = VISA Close(VISA resource name=w275, error in (no error)=w271) -> (error out=w268:errorcluster)
            n147 = Unbundle By Name(w274) -> ("KNF SIMDOS Settings"=w270:T10)
            n148 = call "Initialize.vi"("error in (no error)"=w268, "KNF Settings"=w270) -> ("Initialized"=w264:bool, "KNF Settings"=w269:T10)  [unwired: 6 in, 2 out]
            n149 = case shown="False" w264 {
              tunnel: w269 -> [_ w284]
              tunnel: w273 -> [w279 w283]
              tunnel: [w279 w282] -> w272
              frame False {
                n150 = control-ref of="OK Button"() -> (w277:refnum<vi>)
                n151 = One Button Dialog(message="No Pump Connected") -> ()  [unwired: 1 in, 1 out]
                n152 = property class="Bool"(reference=w277, "DisabledEnum"=T17."Disabled and Grayed Out" ("Disabled")) -> ()  [unwired: 1 in, 2 out]
              }
              frame True {
                n153 = Bundle By Name(cluster=w283, "Settings.KNF SIMDOS Settings"=w284) -> (w282:T2)
                n154 = control-ref of="OK Button"() -> (w280:refnum<vi>)
                n155 = property class="Bool"(reference=w280, "DisabledEnum"=T17."Enabled" ("Disabled")) -> ()  [unwired: 1 in, 2 out]
              }
            }
          }
          event Value Change {
            n156 = event-data() -> ("OldVal"=w296:refnum<visa-resource-name>)  [unwired: 1 in, 5 out]
            n157 = property on="Pump Configuration" class="Clust (strict)"() -> ("Value"=w293:T19)  [unwired: 2 in, 2 out]
            n158 = VISA Close(VISA resource name=w296, error in (no error)=w289) -> (error out=w292:errorcluster)
            n159 = Unbundle By Name(w293) -> ("Masterflex"=w295:T6)
            n160 = call "Initialize.vi"("error in (no error)"=w292, "Masterflex Settings in"=w295) -> ("Initialized"=w285:bool, "Masterflex Settings out"=w294:T6)  [unwired: 6 in, 2 out]
            n161 = case shown="False" w285 {
              tunnel: w294 -> [_ w305]
              tunnel: w291 -> [w300 w304]
              tunnel: [w300 w303] -> w290
              frame False {
                n162 = control-ref of="OK Button"() -> (w298:refnum<vi>)
                n163 = One Button Dialog(message="No Pump Connected") -> ()  [unwired: 1 in, 1 out]
                n164 = property class="Bool"(reference=w298, "DisabledEnum"=T17."Disabled and Grayed Out" ("Disabled")) -> ()  [unwired: 1 in, 2 out]
              }
              frame True {
                n165 = control-ref of="OK Button"() -> (w301:refnum<vi>)
                n166 = Bundle By Name(cluster=w304, "Settings.Masterflex"=w305) -> (w303:T2)
                n167 = property class="Bool"(reference=w301, "DisabledEnum"=T17."Enabled" ("Disabled")) -> ()  [unwired: 1 in, 2 out]
              }
            }
          }
          event Value Change {
            n168 = event-data() -> ("NewVal"=w311:T8)  [unwired: 1 in, 5 out]
            n169 = case "Selected Device" shown="\"KNF SIMDOS\"" w311 {
              tunnel: w310 -> [w319 w330 w341 w351 w363 w374 w383 w403 w414]
              tunnel: [w319 w330 w341 w351 w363 w374 w383 w403 w414] -> w309
              frame "Ismatec ISM 831C" {
                n170 = property on="VICI Settings" class="Clust (strict)"("Visible"=FALSE) -> ()  [unwired: 2 in, 2 out]
                n171 = property on="Tacmina Settings" class="Clust (strict)"("Visible"=FALSE) -> ()  [unwired: 2 in, 2 out]
                n172 = property on="Ismatech" class="Clust (strict)"("Visible"=TRUE) -> ()  [unwired: 2 in, 2 out]
                n173 = property on="Masterflex" class="Clust (strict)"("Visible"=FALSE) -> ()  [unwired: 2 in, 2 out]
                n174 = property on="FLOM Settings" class="Clust (strict)"("Visible"=FALSE) -> ()  [unwired: 2 in, 2 out]
                n175 = property on="KNF SIMDOS Settings" class="Clust (strict)"("Visible"=FALSE) -> ()  [unwired: 2 in, 2 out]
                n176 = property on="ASIA Pump C" class="Clust (strict)"("Visible"=FALSE) -> ()  [unwired: 2 in, 2 out]
                n177 = property on="Pump Calibration" class="Ring (strict)"("Visible"=FALSE) -> ()  [unwired: 2 in, 2 out]
                n178 = property on="SSI PR Settings" class="Clust (strict)"("Visible"=FALSE) -> ()  [unwired: 2 in, 2 out]
                n179 = property on="Pump %" class="DigNum (strict)"("Caption.Text"="Pump %" ("Label.Text")) -> ()  [unwired: 2 in, 2 out]
              }
              frame "Masterflex 7550-30" {
                n180 = property on="VICI Settings" class="Clust (strict)"("Visible"=FALSE) -> ()  [unwired: 2 in, 2 out]
                n181 = property on="Tacmina Settings" class="Clust (strict)"("Visible"=FALSE) -> ()  [unwired: 2 in, 2 out]
                n182 = property on="Ismatech" class="Clust (strict)"("Visible"=FALSE) -> ()  [unwired: 2 in, 2 out]
                n183 = property on="Masterflex" class="Clust (strict)"("Visible"=TRUE) -> ()  [unwired: 2 in, 2 out]
                n184 = property on="FLOM Settings" class="Clust (strict)"("Visible"=FALSE) -> ()  [unwired: 2 in, 2 out]
                n185 = property on="Pump Calibration" class="Ring (strict)"("Visible"=FALSE) -> ()  [unwired: 2 in, 2 out]
                n186 = property on="KNF SIMDOS Settings" class="Clust (strict)"("Visible"=FALSE) -> ()  [unwired: 2 in, 2 out]
                n187 = property on="ASIA Pump C" class="Clust (strict)"("Visible"=FALSE) -> ()  [unwired: 2 in, 2 out]
                n188 = property on="SSI PR Settings" class="Clust (strict)"("Visible"=FALSE) -> ()  [unwired: 2 in, 2 out]
                n189 = property on="Pump %" class="DigNum (strict)"("Caption.Text"="Pump %" ("Label.Text")) -> ()  [unwired: 2 in, 2 out]
              }
              frame "VICI" {
                n190 = property on="Tacmina Settings" class="Clust (strict)"("Visible"=FALSE) -> ()  [unwired: 2 in, 2 out]
                n191 = property on="VICI Settings" class="Clust (strict)"("Visible"=TRUE) -> ()  [unwired: 2 in, 2 out]
                n192 = property on="Ismatech" class="Clust (strict)"("Visible"=FALSE) -> ()  [unwired: 2 in, 2 out]
                n193 = property on="Masterflex" class="Clust (strict)"("Visible"=FALSE) -> ()  [unwired: 2 in, 2 out]
                n194 = property on="KNF SIMDOS Settings" class="Clust (strict)"("Visible"=FALSE) -> ()  [unwired: 2 in, 2 out]
                n195 = property on="ASIA Pump C" class="Clust (strict)"("Visible"=FALSE) -> ()  [unwired: 2 in, 2 out]
                n196 = property on="FLOM Settings" class="Clust (strict)"("Visible"=FALSE) -> ()  [unwired: 2 in, 2 out]
                n197 = property on="Pump Calibration" class="Ring (strict)"("Visible"=TRUE) -> ()  [unwired: 2 in, 2 out]
                n198 = property on="SSI PR Settings" class="Clust (strict)"("Visible"=FALSE) -> ()  [unwired: 2 in, 2 out]
                n199 = property on="Pump %" class="DigNum (strict)"("Caption.Text"="ml/min" ("Label.Text")) -> ()  [unwired: 2 in, 2 out]
              }
              frame "Tacmina QI" {
                n200 = property on="Tacmina Settings" class="Clust (strict)"("Visible"=TRUE) -> ()  [unwired: 2 in, 2 out]
                n201 = property on="VICI Settings" class="Clust (strict)"("Visible"=FALSE) -> ()  [unwired: 2 in, 2 out]
                n202 = property on="Ismatech" class="Clust (strict)"("Visible"=FALSE) -> ()  [unwired: 2 in, 2 out]
                n203 = property on="Masterflex" class="Clust (strict)"("Visible"=FALSE) -> ()  [unwired: 2 in, 2 out]
                n204 = property on="FLOM Settings" class="Clust (strict)"("Visible"=FALSE) -> ()  [unwired: 2 in, 2 out]
                n205 = property on="Pump Calibration" class="Ring (strict)"("Visible"=FALSE) -> ()  [unwired: 2 in, 2 out]
                n206 = property on="KNF SIMDOS Settings" class="Clust (strict)"("Visible"=FALSE) -> ()  [unwired: 2 in, 2 out]
                n207 = property on="ASIA Pump C" class="Clust (strict)"("Visible"=FALSE) -> ()  [unwired: 2 in, 2 out]
                n208 = property on="SSI PR Settings" class="Clust (strict)"("Visible"=FALSE) -> ()  [unwired: 2 in, 2 out]
                n209 = property on="Pump %" class="DigNum (strict)"("Caption.Text"="Pump %" ("Label.Text")) -> ()  [unwired: 2 in, 2 out]
              }
              frame "Default", Default {
                n210 = property on="Tacmina Settings" class="Clust (strict)"("Visible"=FALSE) -> ()  [unwired: 2 in, 2 out]
                n211 = property on="VICI Settings" class="Clust (strict)"("Visible"=FALSE) -> ()  [unwired: 2 in, 2 out]
                n212 = property on="Ismatech" class="Clust (strict)"("Visible"=FALSE) -> ()  [unwired: 2 in, 2 out]
                n213 = property on="Masterflex" class="Clust (strict)"("Visible"=FALSE) -> ()  [unwired: 2 in, 2 out]
                n214 = property on="FLOM Settings" class="Clust (strict)"("Visible"=FALSE) -> ()  [unwired: 2 in, 2 out]
                n215 = property on="KNF SIMDOS Settings" class="Clust (strict)"("Visible"=FALSE) -> ()  [unwired: 2 in, 2 out]
                n216 = property on="ASIA Pump C" class="Clust (strict)"("Visible"=FALSE) -> ()  [unwired: 2 in, 2 out]
                n217 = property on="Pump Calibration" class="Ring (strict)"("Visible"=FALSE) -> ()  [unwired: 2 in, 2 out]
                n218 = property on="SSI PR Settings" class="Clust (strict)"("Visible"=FALSE) -> ()  [unwired: 2 in, 2 out]
                n219 = property on="Pump %" class="DigNum (strict)"("Caption.Text"="Pump %" ("Label.Text")) -> ()  [unwired: 2 in, 2 out]
              }
              frame "KNF SIMDOS" {
                n220 = property on="Tacmina Settings" class="Clust (strict)"("Visible"=FALSE) -> ()  [unwired: 2 in, 2 out]
                n221 = property on="VICI Settings" class="Clust (strict)"("Visible"=FALSE) -> ()  [unwired: 2 in, 2 out]
                n222 = property on="Ismatech" class="Clust (strict)"("Visible"=FALSE) -> ()  [unwired: 2 in, 2 out]
                n223 = property on="Masterflex" class="Clust (strict)"("Visible"=FALSE) -> ()  [unwired: 2 in, 2 out]
                n224 = property on="FLOM Settings" class="Clust (strict)"("Visible"=FALSE) -> ()  [unwired: 2 in, 2 out]
                n225 = property on="KNF SIMDOS Settings" class="Clust (strict)"("Visible"=TRUE) -> ()  [unwired: 2 in, 2 out]
                n226 = property on="ASIA Pump C" class="Clust (strict)"("Visible"=FALSE) -> ()  [unwired: 2 in, 2 out]
                n227 = property on="Pump Calibration" class="Ring (strict)"("Visible"=FALSE) -> ()  [unwired: 2 in, 2 out]
                n228 = property on="SSI PR Settings" class="Clust (strict)"("Visible"=FALSE) -> ()  [unwired: 2 in, 2 out]
                n229 = property on="Pump %" class="DigNum (strict)"("Caption.Text"="Pump %" ("Label.Text")) -> ()  [unwired: 2 in, 2 out]
              }
              frame "ASIA Type C" {
                n230 = Unbundle By Name(w383) -> ("Settings.ASIA Pump C.ASIA Pump #"=w382:i32)
                n231 = property on="Tacmina Settings" class="Clust (strict)"("Visible"=FALSE) -> ()  [unwired: 2 in, 2 out]
                n232 = property on="VICI Settings" class="Clust (strict)"("Visible"=FALSE) -> ()  [unwired: 2 in, 2 out]
                n233 = property on="Ismatech" class="Clust (strict)"("Visible"=FALSE) -> ()  [unwired: 2 in, 2 out]
                n234 = property on="Masterflex" class="Clust (strict)"("Visible"=FALSE) -> ()  [unwired: 2 in, 2 out]
                n235 = property on="KNF SIMDOS Settings" class="Clust (strict)"("Visible"=FALSE) -> ()  [unwired: 2 in, 2 out]
                n236 = property on="ASIA Pump C" class="Clust (strict)"("Visible"=TRUE) -> ()  [unwired: 2 in, 2 out]
                n237 = property on="FLOM Settings" class="Clust (strict)"("Visible"=FALSE) -> ()  [unwired: 2 in, 2 out]
                n238 = property on="Pump Calibration" class="Ring (strict)"("Visible"=FALSE) -> ()  [unwired: 2 in, 2 out]
                n239 = Greater Or Equal To 0?(x=w382) -> (x >= 0?=w381:bool)
                n240 = case shown="False" w381 {
                  frame False {
                    n241 = property on="OK Button" class="Bool"("DisabledEnum"=T17."Disabled and Grayed Out" ("Disabled")) -> ()  [unwired: 2 in, 2 out]
                  }
                  frame True {
                    n242 = property on="OK Button" class="Bool"("DisabledEnum"=T17."Enabled" ("Disabled")) -> ()  [unwired: 2 in, 2 out]
                  }
                }
                n243 = property on="SSI PR Settings" class="Clust (strict)"("Visible"=FALSE) -> ()  [unwired: 2 in, 2 out]
                n244 = property on="Pump %" class="DigNum (strict)"("Caption.Text"="ml/min" ("Label.Text")) -> ()  [unwired: 2 in, 2 out]
              }
              frame "FLOM UI-22-11" {
                n245 = property on="Tacmina Settings" class="Clust (strict)"("Visible"=FALSE) -> ()  [unwired: 2 in, 2 out]
                n246 = property on="VICI Settings" class="Clust (strict)"("Visible"=FALSE) -> ()  [unwired: 2 in, 2 out]
                n247 = property on="Ismatech" class="Clust (strict)"("Visible"=FALSE) -> ()  [unwired: 2 in, 2 out]
                n248 = property on="Masterflex" class="Clust (strict)"("Visible"=FALSE) -> ()  [unwired: 2 in, 2 out]
                n249 = property on="Pump Calibration" class="Ring (strict)"("Visible"=FALSE) -> ()  [unwired: 2 in, 2 out]
                n250 = property on="KNF SIMDOS Settings" class="Clust (strict)"("Visible"=FALSE) -> ()  [unwired: 2 in, 2 out]
                n251 = property on="ASIA Pump C" class="Clust (strict)"("Visible"=FALSE) -> ()  [unwired: 2 in, 2 out]
                n252 = property on="FLOM Settings" class="Clust (strict)"("Visible"=TRUE) -> ()  [unwired: 2 in, 2 out]
                n253 = property on="SSI PR Settings" class="Clust (strict)"("Visible"=FALSE) -> ()  [unwired: 2 in, 2 out]
                n254 = property on="Pump %" class="DigNum (strict)"("Caption.Text"="ml/min" ("Label.Text")) -> ()  [unwired: 2 in, 2 out]
              }
              frame "SSI PR" {
                n255 = property on="VICI Settings" class="Clust (strict)"("Visible"=FALSE) -> ()  [unwired: 2 in, 2 out]
                n256 = property on="Tacmina Settings" class="Clust (strict)"("Visible"=FALSE) -> ()  [unwired: 2 in, 2 out]
                n257 = property on="Ismatech" class="Clust (strict)"("Visible"=FALSE) -> ()  [unwired: 2 in, 2 out]
                n258 = property on="Masterflex" class="Clust (strict)"("Visible"=FALSE) -> ()  [unwired: 2 in, 2 out]
                n259 = property on="FLOM Settings" class="Clust (strict)"("Visible"=FALSE) -> ()  [unwired: 2 in, 2 out]
                n260 = property on="KNF SIMDOS Settings" class="Clust (strict)"("Visible"=FALSE) -> ()  [unwired: 2 in, 2 out]
                n261 = property on="ASIA Pump C" class="Clust (strict)"("Visible"=FALSE) -> ()  [unwired: 2 in, 2 out]
                n262 = property on="Pump Calibration" class="Ring (strict)"("Visible"=FALSE) -> ()  [unwired: 2 in, 2 out]
                n263 = property on="SSI PR Settings" class="Clust (strict)"("Visible"=TRUE) -> ()  [unwired: 2 in, 2 out]
                n264 = property on="Pump %" class="DigNum (strict)"("Caption.Text"="ml/min" ("Label.Text")) -> ()  [unwired: 2 in, 2 out]
              }
            }
          }
          event Value Change {
            n265 = event-data() -> ()  [unwired: 1 in, 6 out]
            n266 = property on="Pump Configuration" class="Clust (strict)"() -> ("Value"=w423:T19)  [unwired: 2 in, 2 out]
            n267 = Unbundle By Name(w423) -> ("SSI PR Settings"=w424:T13)
            n268 = call "Initialize.vi"("error in (no error)"=w420, "SSI PR Settings In"=w424) -> ("Initialized"=w415:bool, "SSI PR Settings Out"=w416:T13)  [unwired: 6 in, 2 out]
            n269 = case shown="False" w415 {
              tunnel: w416 -> [_ w433]
              tunnel: w422 -> [w428 w432]
              tunnel: [w428 w431] -> w421
              frame False {
                n270 = control-ref of="OK Button"() -> (w426:refnum<vi>)
                n271 = One Button Dialog(message="No Pump Connected") -> ()  [unwired: 1 in, 1 out]
                n272 = property class="Bool"(reference=w426, "DisabledEnum"=T17."Disabled and Grayed Out" ("Disabled")) -> ()  [unwired: 1 in, 2 out]
              }
              frame True {
                n273 = Bundle By Name(cluster=w432, "Settings.SSI PR Settings"=w433) -> (w431:T2)
                n274 = control-ref of="OK Button"() -> (w429:refnum<vi>)
                n275 = property class="Bool"(reference=w429, "DisabledEnum"=T17."Enabled" ("Disabled")) -> ()  [unwired: 1 in, 2 out]
              }
            }
          }
          event Value Change {
            n276 = event-data() -> ()  [unwired: 1 in, 6 out]
            n277 = property on="Pump Configuration" class="Clust (strict)"() -> ("Value"=w440:T19)  [unwired: 2 in, 2 out]
            n278 = Unbundle By Name(w440) -> ("Tacmina Settings"=w437:T9)
            n279 = call "Initialize.vi"("Tacmina Settings in"=w437) -> ("Tacmina Settings out"=w441:T9)  [unwired: 8 in, 2 out]
            n280 = Bundle By Name(cluster=w439, "Settings.Tacmina Settings"=w441) -> (w438:T2)
          }
          event Value Change {
            n281 = event-data() -> ()  [unwired: 1 in, 1 out]
            n282 = property on="Pump Configuration" class="Clust (strict)"() -> ("Value"=w448:T19)  [unwired: 2 in, 2 out]
            n283 = Unbundle By Name(w448) -> ("VICI Settings"=w449:T18)
            n284 = case shown="True" w444 {
              tunnel: w449 -> [_ w456]
              tunnel: w447 -> [w450 w454]
              tunnel: [w450 w453] -> w446
              tunnel: w445 -> [_ w452]
              frame False {
              }
              frame True {
                n285 = call "Initialize.vi"("error in (no error)"=w452, "VICI Settings"=w456) -> ("Initialized"=w451:bool, "VICI Settings"=w455:T7)  [unwired: 6 in, 2 out]
                n286 = case shown="False" w451 {
                  tunnel: w455 -> [_ w465]
                  tunnel: w454 -> [w460 w464]
                  tunnel: [w460 w463] -> w453
                  frame False {
                    n287 = control-ref of="OK Button"() -> (w458:refnum<vi>)
                    n288 = One Button Dialog(message="No Pump Connected") -> ()  [unwired: 1 in, 1 out]
                    n289 = property class="Bool"(reference=w458, "DisabledEnum"=T17."Disabled and Grayed Out" ("Disabled")) -> ()  [unwired: 1 in, 2 out]
                  }
                  frame True {
                    n290 = Bundle By Name(cluster=w464, "Settings.VICI Settings"=w465) -> (w463:T2)
                    n291 = control-ref of="OK Button"() -> (w461:refnum<vi>)
                    n292 = property class="Bool"(reference=w461, "DisabledEnum"=T17."Enabled" ("Disabled")) -> ()  [unwired: 1 in, 2 out]
                  }
                }
              }
            }
          }
          event Value Change {
            n293 = event-data() -> ("NewVal"=w466:bool)  [unwired: 1 in, 5 out]
            n294 = case shown="True" w466 {
              frame False {
              }
              frame True {
                n295 = control-ref of="OK Button"() -> (w472:refnum<vi>)
                n296 = property class="Bool"(reference=w472, "DisabledEnum"=T17."Enabled" ("Disabled")) -> ()  [unwired: 1 in, 2 out]
              }
            }
          }
          event Value Change {
            n297 = event-data() -> ("OldVal"=w479:refnum<visa-resource-name>)  [unwired: 1 in, 5 out]
            n298 = property on="Pump Configuration" class="Clust (strict)"() -> ("Value"=w480:T19)  [unwired: 2 in, 2 out]
            n299 = VISA Close(VISA resource name=w479, error in (no error)=w476) -> (error out=w481:errorcluster)
            n300 = Unbundle By Name(w480) -> ("VICI Settings"=w482:T18)
            n301 = case shown="True" w475 {
              tunnel: w482 -> [_ w489]
              tunnel: w481 -> [_ w487]
              tunnel: w478 -> [w483 w486]
              tunnel: [w483 w485] -> w477
              frame False {
              }
              frame True {
                n302 = call "Initialize.vi"("error in (no error)"=w487, "VICI Settings"=w489) -> ("Initialized"=w484:bool, "VICI Settings"=w488:T7)  [unwired: 6 in, 2 out]
                n303 = case shown="False" w484 {
                  tunnel: w488 -> [_ w498]
                  tunnel: w486 -> [w493 w497]
                  tunnel: [w493 w496] -> w485
                  frame False {
                    n304 = control-ref of="OK Button"() -> (w491:refnum<vi>)
                    n305 = property class="Bool"(reference=w491, "DisabledEnum"=T17."Disabled and Grayed Out" ("Disabled")) -> ()  [unwired: 1 in, 2 out]
                    n306 = One Button Dialog(message="No Pump Connected") -> ()  [unwired: 1 in, 1 out]
                  }
                  frame True {
                    n307 = Bundle By Name(cluster=w497, "Settings.VICI Settings"=w498) -> (w496:T2)
                    n308 = control-ref of="OK Button"() -> (w494:refnum<vi>)
                    n309 = property class="Bool"(reference=w494, "DisabledEnum"=T17."Enabled" ("Disabled")) -> ()  [unwired: 1 in, 2 out]
                  }
                }
              }
            }
          }
          event "Pump Settings.Start": Value Change {
            n310 = event-data() -> ()  [unwired: 1 in, 6 out]
            n311 = control-ref of="Start"() -> (w504:refnum<vi>)
            n312 = control-ref of="Stop"() -> (w503:refnum<vi>)
            n313 = Build Array(w504) -> (w506:refnum<vi>[])
            n314 = Build Array(w503) -> (w508:refnum<vi>[])
            n315 = call "Set Enable State on Multiple Controls.vi"("Enable?"=FALSE, "Controls"=w506) -> ()  [unwired: 10 in]
            n316 = call "Set Enable State on Multiple Controls.vi"("Enable?"=TRUE, "Controls"=w508) -> ()  [unwired: 10 in]
          }
          event "Pump Settings.Stop": Value Change {
            n317 = event-data() -> ()  [unwired: 1 in, 6 out]
            n318 = control-ref of="Start"() -> (w514:refnum<vi>)
            n319 = control-ref of="Stop"() -> (w513:refnum<vi>)
            n320 = Build Array(w514) -> (w518:refnum<vi>[])
            n321 = Build Array(w513) -> (w516:refnum<vi>[])
            n322 = call "Set Enable State on Multiple Controls.vi"("Enable?"=TRUE, "Controls"=w518) -> ()  [unwired: 10 in]
            n323 = call "Set Enable State on Multiple Controls.vi"("Enable?"=FALSE, "Controls"=w516) -> ()  [unwired: 10 in]
          }
          event Value Change {
            n324 = event-data() -> ("NewVal"=w520:bool)  [unwired: 1 in, 5 out]
            n325 = Equal?(x=w520, y=TRUE) -> (x = y?=w519:bool)
            n326 = case shown="True" w519 {
              frame False {
              }
              frame True {
                n327 = property on="OK Button" class="Bool"("DisabledEnum"=T17."Enabled" ("Disabled")) -> ()  [unwired: 2 in, 2 out]
              }
            }
          }
        }
      }
      n328 = case shown="True" w23 {
        tunnel: w22 -> [w527 w528]
        tunnel: [_ w529] -> w31
        tunnel: [w527 w528] -> w32
        frame False {
        }
        frame True {
          # "Write settings back to XML"
          n329 = Flatten To XML(anything=w528) -> (xml string=w530:string)
          n330 = call "Get Config File Path.vi"() -> ("XML File Path"=w531:path)  [unwired: 10 in, 1 out]
          n331 = call-poly <vilib>:"Write to XML File.vi"("XML Input"=w530, "XML File Path"=w531) -> ("error out"=w529:errorcluster)  [unwired: 7 in, 2 out]
        }
      }
    }
    frame Error {
    }
  }
  "UI Refresh Needed?" <- w12
  "error out" <- w13
  "Cancelled?" <- w11
  "Pump Module Config Out" <- w7
